vi "Test - Merge JSON - Object.vi"() -> (0 "error out":errorcluster)   [LabVIEW 2020, in "JSON Schema Generator.lvlib"]
uses:
  JSON Schema Generator.lvlib
  <vilib>/addons/_JKI Toolkits/Caraya/classes/Test/Test.lvclass
  <vilib>/addons/_JKI Toolkits/Caraya/classes/Assert/Assert.lvclass
  <vilib>/addons/_JKI Toolkits/Caraya/classes/Assert/Assert Not Error.vi
  <vilib>/addons/_JKI Toolkits/Caraya/classes/Assert/Assert Equal Value_Variant.vi
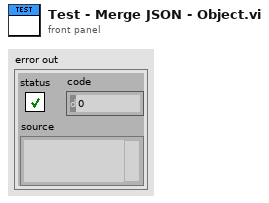
[diagram p1: front panel]
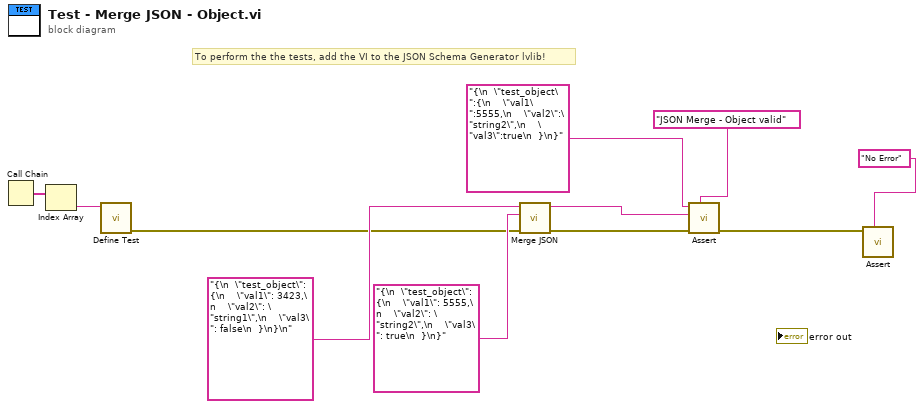
[diagram p0: block diagram]
diagram:
  # "To perform the the tests, add the VI to the JSON Schema Generator lvlib!"
  n1 = Call Chain() -> (call chain=w11:string[])
  n2 = Index Array(array=w11) -> (element=w10:string)  [unwired: 1 in]
  n3 = call <vilib>:"Define Test.vi"("Label (VI Title)"=w10) -> ("error out"=w3:errorcluster)  [unwired: 9 in, 1 out]
  n4 = call "Merge JSON.vi"("error in (no error)"=w3, "<JSON> to merge in"="{\n  \"test_object\": {\n    \"val1\": 5555,\n    \"val2\": \"string2\",\n    \"val3\": true\n  }\n}", "<JSON> in"="{\n  \"test_object\": {\n    \"val1\": 3423,\n    \"val2\": \"string1\",\n    \"val3\": false\n  }\n}\n") -> ("error out"=w8:errorcluster, "<JSON> out"=w4:string)  [unwired: 7 in]
  n5 = call-poly <vilib>:"Assert.vi"("Label"="JSON Merge - Object valid", "error in (no error)"=w8, "Actual"=w4, "Expected"="{\n  \"test_object\":{\n    \"val1\":5555,\n    \"val2\":\"string2\",\n    \"val3\":true\n  }\n}" ("<JSON> in")) -> ("error out"=w9:errorcluster)  [unwired: 6 in, 1 out]
  n6 = call-poly <vilib>:"Assert.vi"("Label"="No Error", "Not Error?"=w9) -> ()  [unwired: 8 in, 2 out]
